vi "Read files T(Delay).vi"(10 "Path":path, 11 "Number":dbl) -> (3 "Time":dbl format="%_1g")   [LabVIEW 2020, in "GPP.lvlib"]
uses:
  GPP.lvlib
panel:
  out "String":string
  out "String 2":string
  out "String 3":string
  out "Array":u8[](array[numeric])
  out "Numeric":u16
  out "T1":string
  out "Time":string
  out "LAST1":string
  out "Voltege":string
  out "ALL":string
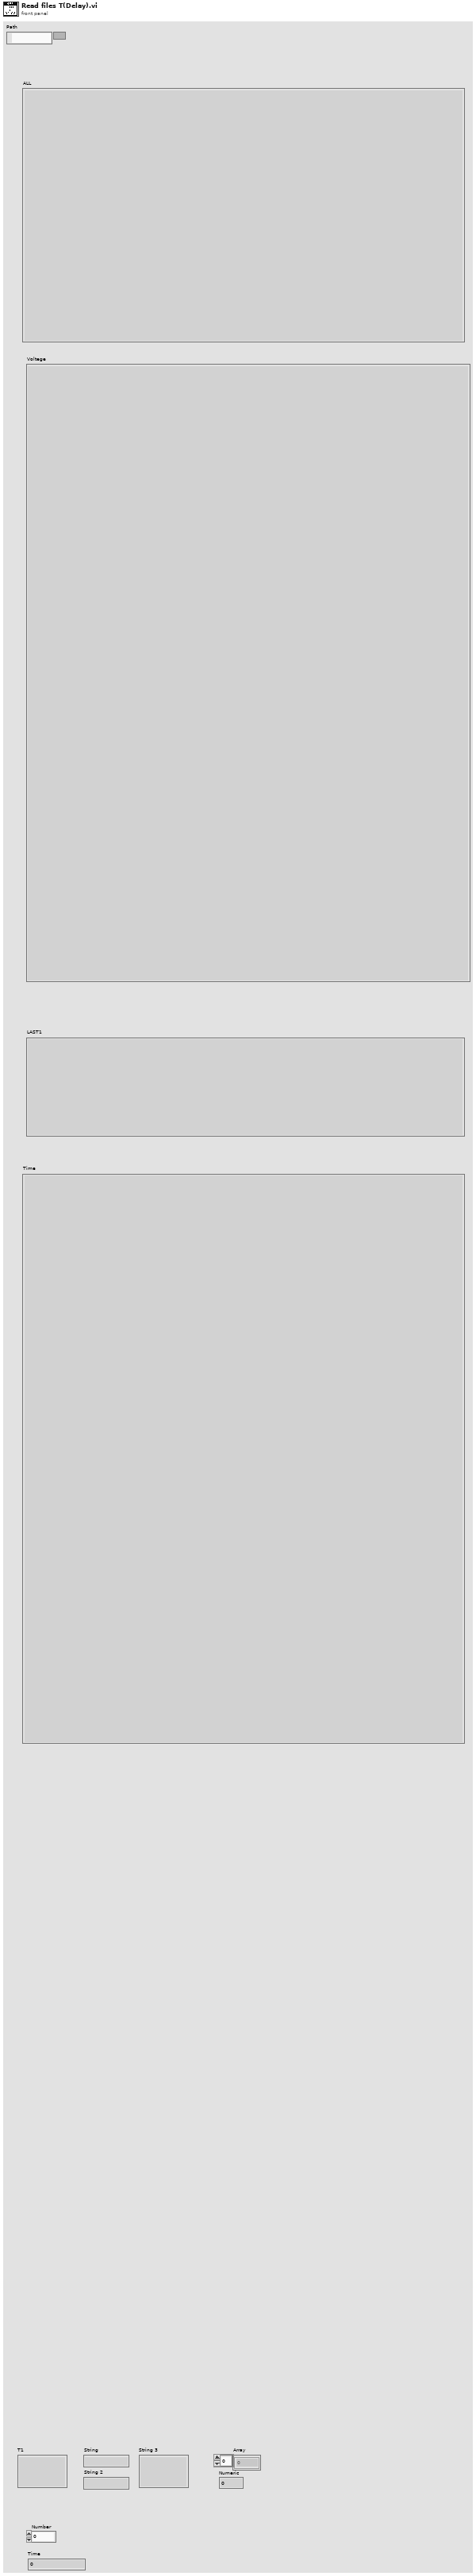
[diagram p1: front panel]
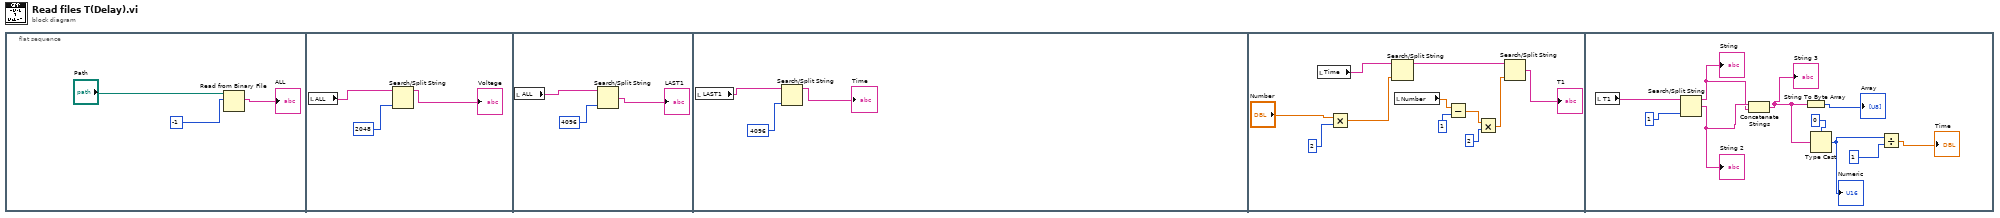
[diagram p0: block diagram]
diagram:
  n1 = flat-sequence {
    frame #0 {
      n2 = Read from Binary File(10:-1, 11:"Path") -> (2:→"ALL":string)  [unwired: 4 in, 3 out]
    }
    frame #1 {
      n3 = local read "ALL"() -> (w4:string)
      n4 = Search/Split String(string=w4, offset (0)=2048) -> (substring before match=→"Voltege":string)  [unwired: 1 in, 2 out]
    }
    frame #2 {
      n5 = local read "ALL"() -> (w7:string)
      n6 = Search/Split String(string=w7, offset (0)=4096) -> (match + rest of string=→"LAST1":string)  [unwired: 1 in, 2 out]
    }
    frame #3 {
      n7 = local read "LAST1"() -> (w10:string)
      n8 = Search/Split String(string=w10, offset (0)=4096) -> (substring before match=→"Time":string)  [unwired: 1 in, 2 out]
    }
    frame #4 {
      n9 = local read "Time"() -> (w13:string)
      n10 = Multiply(x="Number", y=2) -> (x*y=w16:dbl)
      n11 = Search/Split String(string=w13, offset (0)=w16) -> (substring before match=w17:string)  [unwired: 1 in, 2 out]
      n12 = local read "Number"() -> (w19:dbl)
      n13 = Subtract(x=w19, y=1) -> (x-y=w20:dbl)
      n14 = Multiply(x=w20, y=2) -> (x*y=w22:dbl)
      n15 = Search/Split String(string=w17, offset (0)=w22) -> (match + rest of string=→"T1":string)  [unwired: 1 in, 2 out]
    }
    frame #5 {
      n16 = local read "T1"() -> (w24:string)
      n17 = Search/Split String(string=w24, offset (0)=1) -> (substring before match=w26:string, match + rest of string=w27:string)  [unwired: 1 in, 1 out]
      "String" <- w26
      "String 2" <- w27
      n18 = Concatenate Strings(w27, w26) -> (w29:string)
      "String 3" <- w29
      n19 = String To Byte Array(string=w29) -> (unsigned byte array=→"Array":u8[])
      n20 = Type Cast(type=u16 0, x=w29) -> (*(type *) &x=w31:u16)
      "Numeric" <- w31
      n21 = Divide(x=w31, y=1) -> (x/y=→"Time":dbl)
    }
  }
